vi "Cursor.Manage.vi"(8 "error in (no error)":errorcluster, 11 "Cmd list":string[](array[string])) -> (0 "error out":errorcluster)   [LabVIEW 2013, in "Simple Sequence Editor.lvlib"]
uses:
  Simple Sequence Editor.lvlib
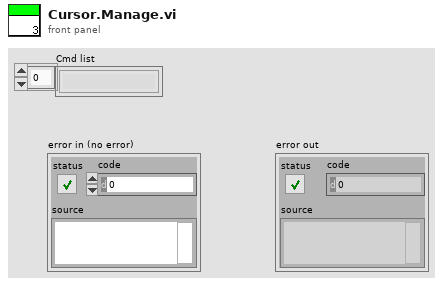
[diagram p1: front panel]
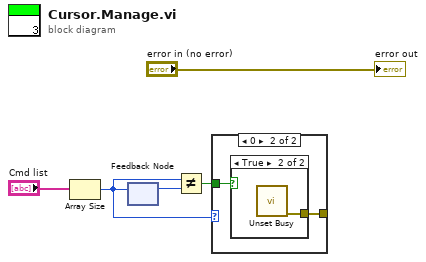
[diagram p0: block diagram]
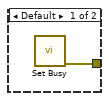
[diagram p2: hidden frame]
diagram:
  n1 = Array Size(array="Cmd list") -> (size(s)=w3:i32)
  n2 = feedback #1(w3) -> (w4:i32)
  n3 = feedback-in #1(w3) -> ()
  n4 = Not Equal?(x=w3, y=w4) -> (x != y?=w2:bool)
  n5 = case shown="0" w3 {
    tunnel: w2 -> [_ w8]
    tunnel: [w6 w7] -> _
    frame Default {
      n6 = call <vilib>:"Set Busy.vi"() -> ("error out"=w6:errorcluster)  [unwired: 10 in, 1 out]
    }
    frame 0 {
      n7 = case shown="True" w8 {
        tunnel: [_ w9] -> w7
        frame False {
        }
        frame True {
          n8 = call <vilib>:"Unset Busy.vi"() -> ("error out"=w9:errorcluster)  [unwired: 11 in]
        }
      }
    }
  }
  "error out" <- "error in (no error)"
